vi "ATDome_logEvent_internalCommand.vi"(8 "error in (no error)":errorcluster, 11 "logevent_internalCommand_Ctl":T1) -> (0 "error out":errorcluster, 2 "function return":i32, 3 "logevent_internalCommand_Ctl out":T1)   [LabVIEW 2016, in "SALLV_ATDome.lvlib"]
doc: "int ATDome_shm_logEvent_internalCommandLV(ATDome_logevent_internalCommandLV *logevent_internalCommand_Ctl );"
uses:
  SALLV_ATDome.lvlib
  DataTypes/logevent_internalCommand.ctl
  SALLV_ATDome.so
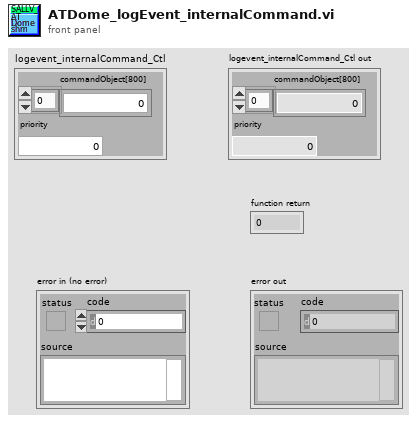
[diagram p1: front panel]
types:
  T1 = typedef "SALLV_ATDome.lvlib/logevent_internalCommand.ctl" = cluster{"commandObject[800]":u8[], "priority":i32}
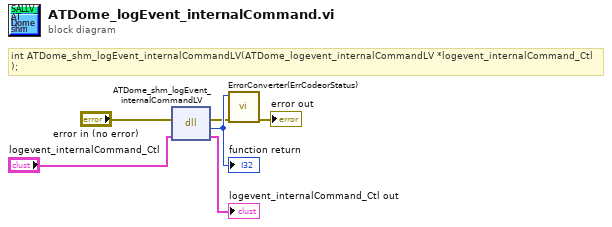
[diagram p0: block diagram]
diagram:
  # "int ATDome_shm_logEvent_internalCommandLV(ATDome_logevent_internalCommandLV *logevent_internalCommand_Ctl );"
  n1 = dll-call lib="home/andres/Desktop/SAL_ATDome/SALLV_ATDome.*" fn="ATDome_shm_logEvent_internalCommandLV"(error in="error in (no error)", "logevent_internalCommand_Ctl"="logevent_internalCommand_Ctl") -> (error out=w2:errorcluster, w6:i32, "logevent_internalCommand_Ctl"=→"logevent_internalCommand_Ctl out":T1)  [unwired: 2 in, 1 out]
  "function return" <- w6
  n2 = call "ErrorConverter(ErrCodeorStatus).vi"("error in (no error)"=w2, "error code"=w6) -> ("error out"=→"error out":errorcluster)  [unwired: 9 in]
